vi "MathOptim-Logistic Estimate.vi"(0 "Y":dbl[](array[numeric]), 5 "X":dbl[](array[numeric])) -> (4 "Initial guess":dbl[](array[numeric]))   [LabVIEW 2015]
uses:
  <vilib>/Analysis/baseanly.llb/Mean (DBL).vi
  <vilib>/Analysis/NI_AALBase.lvlib
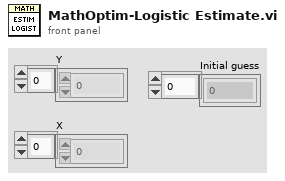
[diagram p1: front panel]
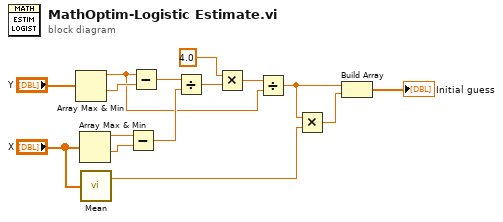
[diagram p0: block diagram]
diagram:
  n1 = Array Max & Min(array="Y") -> (max value=w4:dbl, min value=w10:dbl)  [unwired: 2 out]
  n2 = Array Max & Min(array="X") -> (max value=w12:dbl, min value=w11:dbl)  [unwired: 2 out]
  n3 = call-poly <vilib>:"Mean.vi"("X"="X") -> ("mean"=w2:dbl)  [unwired: 1 out]
  n4 = Subtract(x=w12, y=w11) -> (x-y=w8:dbl)
  n5 = Subtract(x=w4, y=w10) -> (x-y=w9:dbl)
  n6 = Divide(x=w9, y=w8) -> (x/y=w7:dbl)
  n7 = Multiply(x=4.0, y=w7) -> (x*y=w5:dbl)
  n8 = Divide(x=w5, y=w4) -> (x/y=w3:dbl)
  n9 = Multiply(x=w3, y=w2) -> (x*y=w1:dbl)
  n10 = Build Array(w3, w1) -> (→"Initial guess":dbl[])
